vi "TTLReceive.vi"(0 "channel":u16=1 min=1 max=8, 7 "socket in":refnum<class "zmq_socket.lvclass">, 11 "error in":errorcluster) -> (4 "timeout?":bool, 6 "new TTL":bool, 8 "socket out":refnum<class "zmq_socket.lvclass">, 12 "event on":bool, 13 "timestamp":i64, 14 "metadata":string, 15 "error out":errorcluster)   [LabVIEW 2017]
doc: "Attemts to receive one TTL event (non-blocking). If no event is present, then the output \"timeout?\" is true. Otherwise, \"timeout?\" is false and unless an error occurs (such as receiving an event that is not in the TTL format), the other outputs contain the event data."
uses:
  <vilib>/addons/zeromq/zmq_socket.lvclass
  EventBaseType.ctl
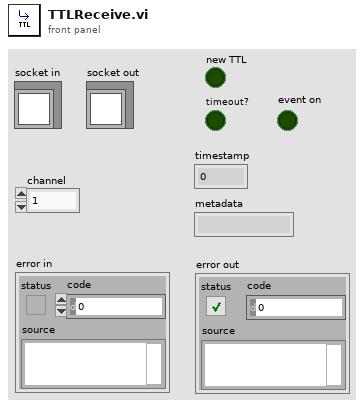
[diagram p1: front panel]
types:
  T1 = enum16{"big-endian, network order", "native, host order", "little-endian"}
  T2 = typedef "EventBaseType.ctl" = enum16{"SYSTEM_EVENT", "PROCESSOR_EVENT", "SPIKE_EVENT"}
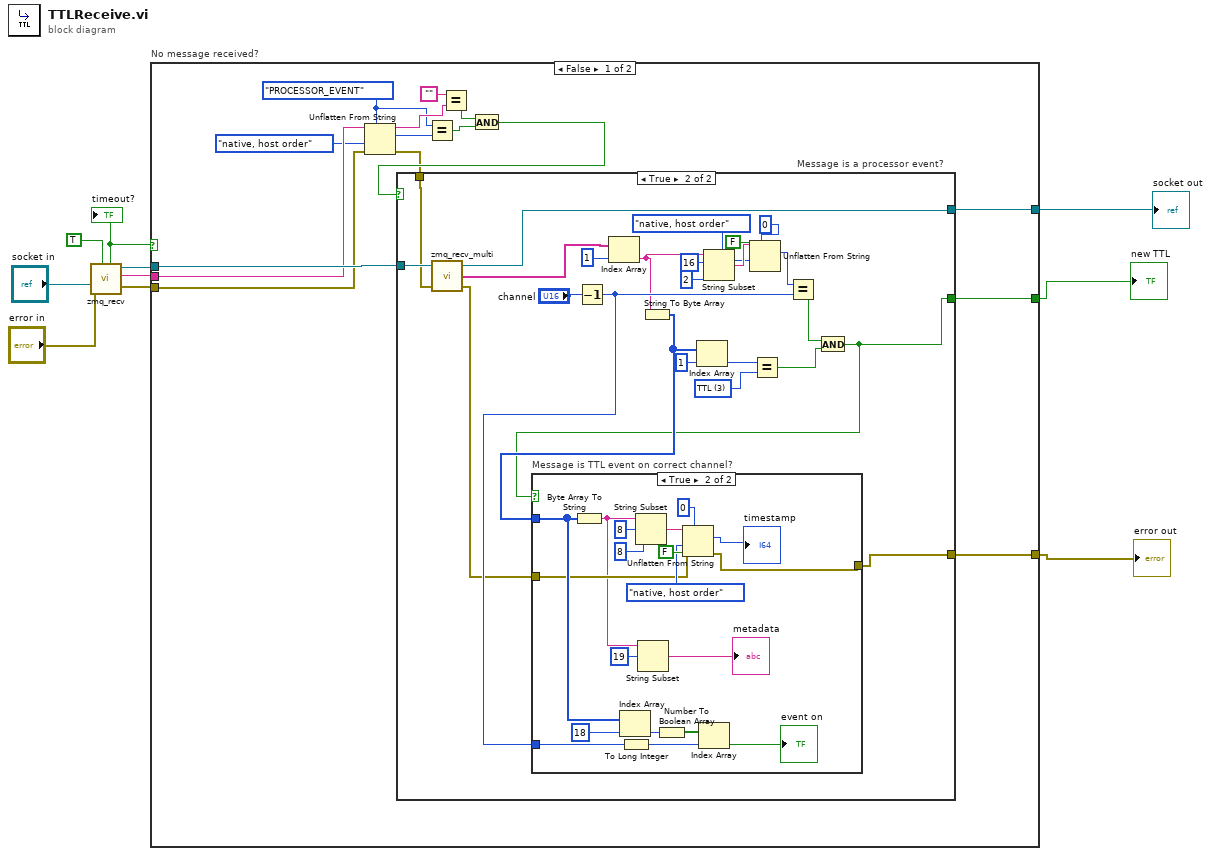
[diagram p0: block diagram]
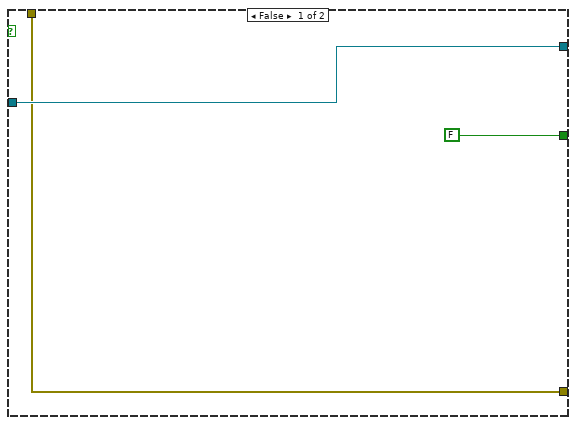
[diagram p2: hidden frame]
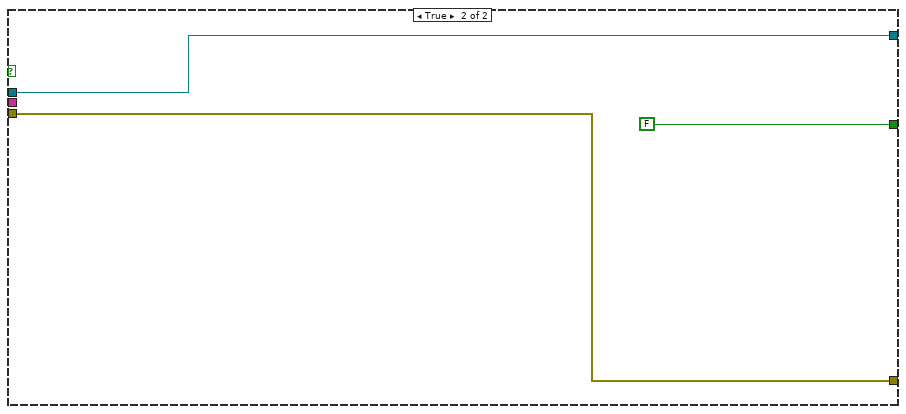
[diagram p4: hidden frame]
diagram:
  n1 = call <vilib>:"zmq_recv.vi"("no block? (F)"=TRUE, "error in"="error in", "socket in"="socket in") -> ("error out"=w4:errorcluster, "data"=w5:string, "socket out"=w6:refnum<class "zmq_socket.lvclass">, "timeout?"=w7:bool)  [unwired: 2 in, 1 out]
  "timeout?" <- w7
  n2 = case "No message received?" shown="False" w7 {
    tunnel: w4 -> [w20 w75]
    tunnel: w6 -> [w25 w74]
    tunnel: w5 -> [w22 _]
    tunnel: [w24 w74] -> w3
    tunnel: [w23 w75] -> w2
    tunnel: [w12 FALSE] -> w1
    frame False {
      w11 = EventBaseType."PROCESSOR_EVENT" ("Event base type")
      n3 = Unflatten From String(type=w11, binary string=w22, byte order (0:big-endian, network order)=T1."native, host order", error in (no error)=w20) -> (rest of the binary string=w17:string, value=w19:T2, error out=w13:errorcluster)  [unwired: 1 in]
      n4 = Equal?(x=w11, y=w19) -> (x = y?=w15:bool)
      n5 = Equal?(x="", y=w17) -> (x = y?=w16:bool)
      n6 = And(x=w16, y=w15) -> (x .and. y?=w14:bool)
      n7 = case "Message is a processor event?" shown="True" w14 {
        tunnel: w25 -> [w28 w52]
        tunnel: [w28 w48] -> w24
        tunnel: [w27 w37] -> w23
        tunnel: w13 -> [w27 w47]
        tunnel: [FALSE w40] -> w12
        frame False {
        }
        frame True {
          w43 = u8 3 items=["TTL"=3, "TEXT"=5, "INT8_ARRAY"=10, "UINT8_ARRAY"=11, "INT16_ARRAY"=12, "UINT16_ARRAY"=13, "INT32_ARRAY"=14, "UINT32_ARRAY"=15, "INT64_ARRAY"=16, "UINT64_ARRAY"=17, "FLOAT_ARRAY"=18, "DOUBLE_ARRAY"=19, "INVALID"=20]
          n8 = call <vilib>:"zmq_recv_multi.vi"("error in"=w47, "socket in"=w52) -> ("error out"=w38:errorcluster, "parts"=w49:string[], "socket out"=w48:refnum<class "zmq_socket.lvclass">)  [unwired: 1 in]
          n9 = Decrement(x="channel") -> (x-1=w39:u16)
          n10 = Index Array(array=w49, index=1) -> (element=w34:string)
          n11 = String To Byte Array(string=w34) -> (unsigned byte array=w46:u8[])
          n12 = Index Array(array=w46, index=1) -> (element=w44:u8)
          n13 = String Subset(string=w34, offset (0)=16, length (rest)=2 ("length (rest)")) -> (substring=w33:string)
          n14 = Unflatten From String(type=u16 0, binary string=w33, data includes array or string size? (T)=FALSE, byte order (0:big-endian, network order)=T1."native, host order") -> (value=w29:u16)  [unwired: 1 in, 2 out]
          n15 = Equal?(x=w44, y=w43) -> (x = y?=w42:bool)
          n16 = Equal?(x=w29, y=w39) -> (x = y?=w41:bool)
          n17 = And(x=w41, y=w42) -> (x .and. y?=w40:bool)
          n18 = case "Message is TTL event on correct channel?" shown="True" w40 {
            tunnel: w46 -> [_ w68]
            tunnel: w39 -> [_ w55]
            tunnel: w38 -> [w53 w60]
            tunnel: [w53 w59] -> w37
            frame False {
            }
            frame True {
              n19 = Byte Array To String(unsigned byte array=w68) -> (string=w58:string)
              n20 = Index Array(array=w68, index=18) -> (element=w71:u8)
              n21 = To Long Integer(number=w55) -> (32bit integer=w54:i32)
              n22 = String Subset(string=w58, offset (0)=8, length (rest)=8 ("length (rest)")) -> (substring=w65:string)
              n23 = String Subset(string=w58, offset (0)=19) -> (substring=→"metadata":string)  [unwired: 1 in]
              n24 = Number To Boolean Array(number=w71) -> (Boolean array=w70:bool[])
              n25 = Unflatten From String(type=i64 0, binary string=w65, data includes array or string size? (T)=FALSE, byte order (0:big-endian, network order)=T1."native, host order", error in (no error)=w60) -> (value=→"timestamp":i64, error out=w59:errorcluster)  [unwired: 1 out]
              n26 = Index Array(array=w70, index=w54) -> (element=→"event on":bool)
            }
          }
        }
      }
    }
    frame True {
    }
  }
  "error out" <- w2
  "socket out" <- w3
  "new TTL" <- w1
